vi "Cryo-Con Get Controls.vi"(8 "error in (no error)":errorcluster, 10 "Control Panel Data":T1={"Channels to measure"=[], "Record heater"=FALSE, "Set point"=0.0, "Heater Range"=enum."0.25W", "Control"=FALSE, "Loop type"=enum."Off", "Ramp rate,\n K/min"=1.0, "Control Channel"="A", "P"=0.0, "I"=0.0, "D"=0.0, "Manual %"=0}, 11 "VISA resource name":refnum<visa-resource-name>) -> (0 "error out":errorcluster, 2 "Control Panel Data Out":T1={"Channels to measure"=[], "Record heater"=FALSE, "Set point"=0.0, "Heater Range"=enum."0.25W", "Control"=FALSE, "Loop type"=enum."Off", "Ramp rate,\n K/min"=1.0, "Control Channel"="A", "P"=0.0, "I"=0.0, "D"=0.0, "Manual %"=0}, 3 "VISA Resource Name Out":refnum<visa-resource-name>)   [LabVIEW 2015]
uses:
  Cryo-Con Front Panel Data.ctl
  Cryo-con Heater Ranges.ctl
  Cry-Con Loop Type.ctl
  GPIB/VISA  Send Receive.vi
panel:
  out "Buffer content":string[](array[string])
  out "data string out":string
  out "data string":string
  # "Temperature Monitor"
  # "Temperature Control"
  # "Temperature Monitor"
  # "Temperature Control"
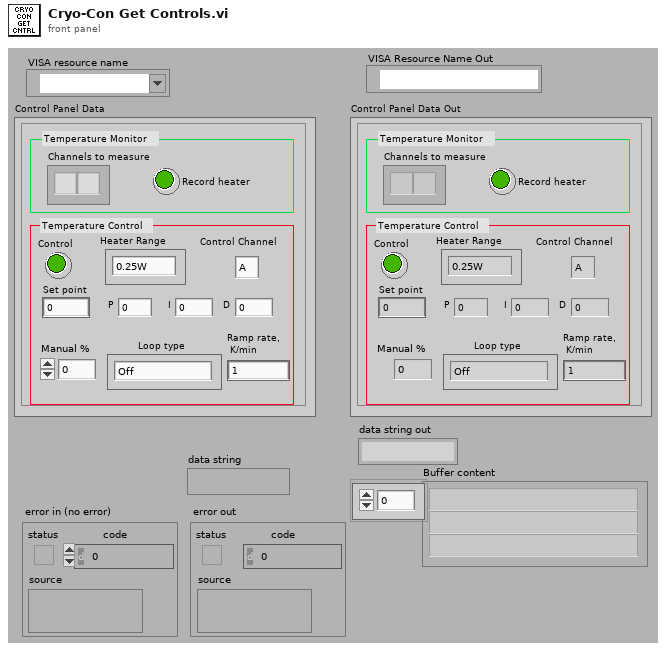
[diagram p1: front panel]
types:
  T1 = typedef "Cryo-Con Front Panel Data.ctl" = cluster{"Channels to measure":string[], "Record heater":bool, "Set point":dbl, "Heater Range":T2, "Control":bool, "Loop type":T3, "Ramp rate,\n K/min":dbl, "Control Channel":string, "P":dbl, "I":dbl, "D":dbl, "Manual %":u16}
  T2 = typedef "Cryo-con Heater Ranges.ctl" = enum16{"25W", "2.5W", "0.25W"}
  T3 = typedef "Cry-Con Loop Type.ctl" = enum16{"Off", "PID", "Manual", "PID Table", "PID Ramp", "PID Table Ramp"}
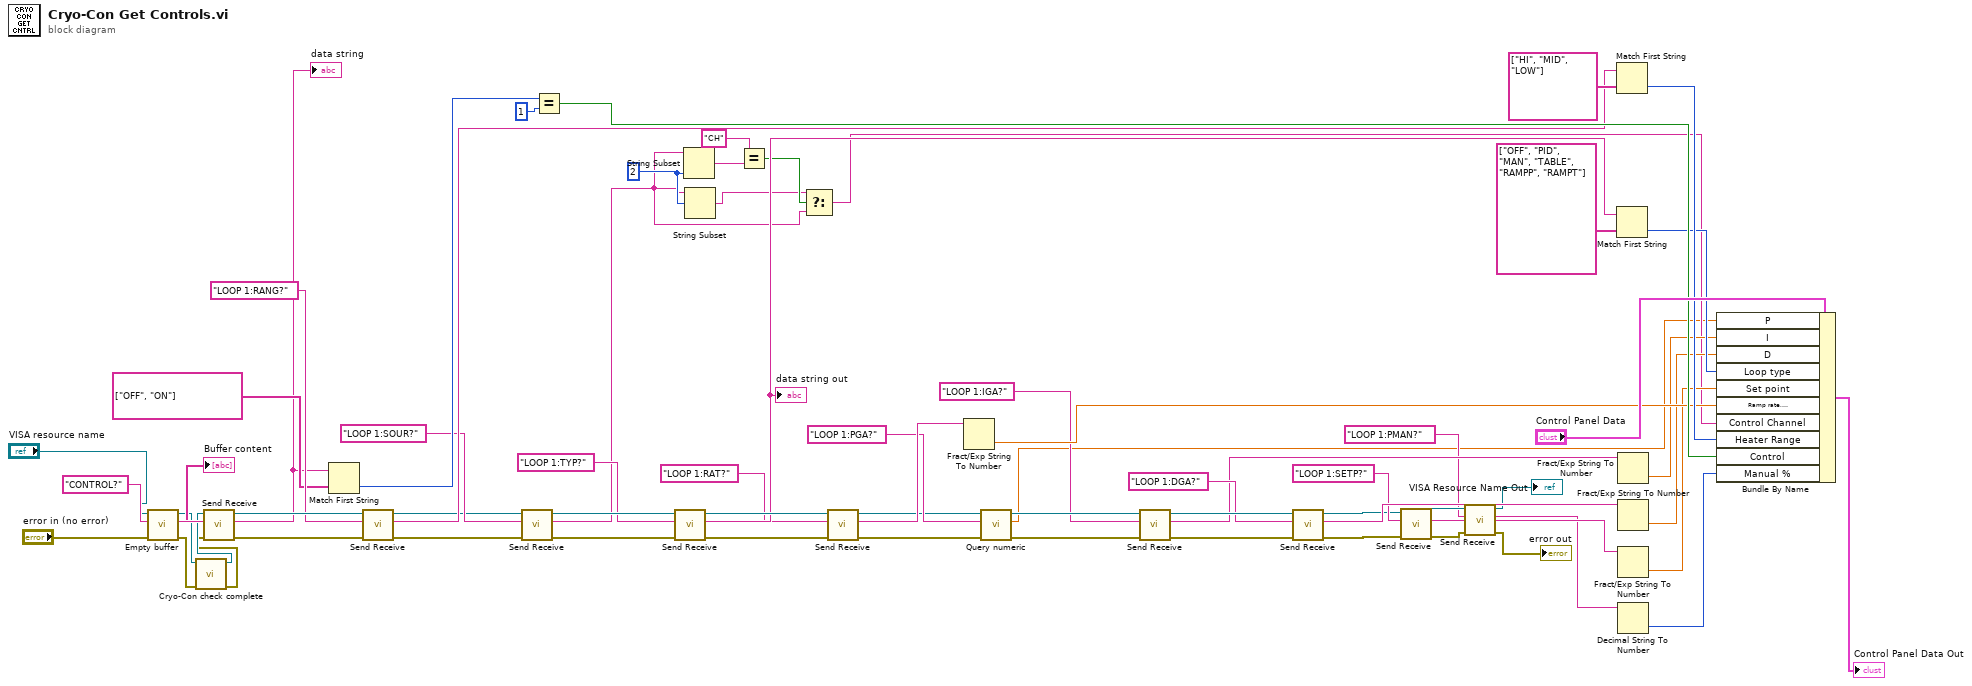
[diagram p0: block diagram]
diagram:
  w22 = 2 ("offset (0)")
  n1 = call "Empty buffer.vi"("Error In"="error in (no error)", "VISA resource name"="VISA resource name") -> ("Error Out"=w3:errorcluster, "Buffer content"=→"Buffer content":string[], "VISA resource name out"=w4:refnum<visa-resource-name>)  [unwired: 7 in]
  n2 = call "Cryo-Con check complete.vi"("Error In"=w3, "VISA resource name"=w4) -> ("Error Out"=w1:errorcluster, "VISA resource name out"=w2:refnum<visa-resource-name>)  [unwired: 8 in]
  n3 = call-poly "Send Receive.vi"("error in (no error)"=w1, "data string in"="CONTROL?" ("data string"), "VISA Resource Name"=w2) -> ("error out"=w58:errorcluster, "data string out"=w59:string, "VISA Resource Name Out"=w63:refnum<visa-resource-name>)  [unwired: 6 in]
  "data string" <- w59
  n4 = Match First String(2:string[] ["OFF", "ON"] ("string array"), 3:w59) -> (0:w57:i32)  [unwired: 1 out]
  n5 = call-poly "Send Receive.vi"("error in (no error)"=w58, "data string in"="LOOP 1:RANG?", "VISA Resource Name"=w63) -> ("error out"=w54:errorcluster, "data string out"=w55:string, "VISA Resource Name Out"=w52:refnum<visa-resource-name>)  [unwired: 6 in]
  n6 = call-poly "Send Receive.vi"("error in (no error)"=w54, "data string in"="LOOP 1:SOUR?", "VISA Resource Name"=w52) -> ("error out"=w49:errorcluster, "data string out"=w17:string, "VISA Resource Name Out"=w51:refnum<visa-resource-name>)  [unwired: 6 in]
  n7 = Equal?(x=w57, y=1) -> (x = y?=w64:bool)
  n8 = call-poly "Send Receive.vi"("error in (no error)"=w49, "data string in"="LOOP 1:TYP?" ("format string"), "VISA Resource Name"=w51) -> ("error out"=w41:errorcluster, "data string out"=w46:string, "VISA Resource Name Out"=w61:refnum<visa-resource-name>)  [unwired: 6 in]
  "data string out" <- w46
  n9 = String Subset(string=w17, length (rest)=w22) -> (substring=w21:string)  [unwired: 1 in]
  n10 = String Subset(string=w17, offset (0)=w22) -> (substring=w18:string)  [unwired: 1 in]
  n11 = Equal?(x="CH", y=w21) -> (x = y?=w19:bool)
  n12 = Select(t=w18, s=w19, f=w17) -> (s? t:f=w16:string)
  n13 = call-poly "Send Receive.vi"("error in (no error)"=w41, "data string in"="LOOP 1:RAT?" ("format string"), "VISA Resource Name"=w61) -> ("error out"=w33:errorcluster, "data string out"=w43:string, "VISA Resource Name Out"=w23:refnum<visa-resource-name>)  [unwired: 6 in]
  n14 = Fract/Exp String To Number(string=w43) -> (number=w42:dbl)  [unwired: 3 in, 1 out]
  n15 = call "Query numeric.vi"("Error In"=w33, "Query String"="LOOP 1:PGA?" ("format string"), "VISA resource name"=w23) -> ("Error Out"=w32:errorcluster, "Numeric"=w8:dbl, "VISA resource name out"=w39:refnum<visa-resource-name>)  [unwired: 5 in, 1 out]
  n16 = call-poly "Send Receive.vi"("error in (no error)"=w32, "data string in"="LOOP 1:IGA?" ("format string"), "VISA Resource Name"=w39) -> ("error out"=w31:errorcluster, "data string out"=w35:string, "VISA Resource Name Out"=w38:refnum<visa-resource-name>)  [unwired: 6 in]
  n17 = call-poly "Send Receive.vi"("error in (no error)"=w31, "data string in"="LOOP 1:DGA?" ("format string"), "VISA Resource Name"=w38) -> ("error out"=w26:errorcluster, "data string out"=w34:string, "VISA Resource Name Out"=w25:refnum<visa-resource-name>)  [unwired: 6 in]
  n18 = call-poly "Send Receive.vi"("error in (no error)"=w26, "data string in"="LOOP 1:SETP?" ("format string"), "VISA Resource Name"=w25) -> ("error out"=w14:errorcluster, "data string out"=w28:string, "VISA Resource Name Out"=w15:refnum<visa-resource-name>)  [unwired: 6 in]
  n19 = call-poly "Send Receive.vi"("error in (no error)"=w14, "data string in"="LOOP 1:PMAN?" ("format string"), "VISA Resource Name"=w15) -> ("error out"=→"error out":errorcluster, "data string out"=w10:string, "VISA Resource Name Out"=→"VISA Resource Name Out":refnum<visa-resource-name>)  [unwired: 6 in]
  n20 = Match First String(2:string[] ["HI", "MID", "LOW"] ("string array"), 3:w55) -> (0:w47:i32)  [unwired: 1 out]
  n21 = Match First String(2:string[] ["OFF", "PID", "MAN", "TABLE", "RAMPP", "RAMPT"] ("string array"), 3:w46) -> (0:w45:i32)  [unwired: 1 out]
  n22 = Fract/Exp String To Number(string=w35) -> (number=w30:dbl)  [unwired: 3 in, 1 out]
  n23 = Fract/Exp String To Number(string=w34) -> (number=w29:dbl)  [unwired: 3 in, 1 out]
  n24 = Fract/Exp String To Number(string=w28) -> (number=w24:dbl)  [unwired: 3 in, 1 out]
  n25 = Decimal String To Number(string=w10) -> (number=w9:i32)  [unwired: 2 in, 1 out]
  n26 = Bundle By Name(cluster="Control Panel Data", "P"=w8, "I"=w30, "D"=w29, "Loop type"=w45, "Set point"=w24, "Ramp rate,\n K/min"=w42, "Control Channel"=w16, "Heater Range"=w47, "Control"=w64, "Manual %"=w9) -> (→"Control Panel Data Out":T1)
